vi "Logger.End.vi"(8 "error in":errorcluster, 10 "SeqData":T1={"BeginTS"=timestamp(0 s since 1904-01-01), "EndTS"=timestamp(0 s since 1904-01-01), "State"=enum."Init", "Status.Work"=enum."-", "Status.Process"=enum."-", "Status.Home"=enum."-", "Status.Wabco"=enum."-", "Status.Client"=enum."-", "BreakReason"=enum."OK container", "BreakSource"=enum."-", "DoorLock"=FALSE, "Status.Prod"=[], "UserAction"={"Stop"=FALSE, "Pause"=FALSE, "Next"=FALSE}, "UserData"={"GuiMode"=enum."Process", "Test"={"IgnoreResults"=FALSE, "IgnoreImages"=FALSE, "ServiceMode"=FALSE}, "ContinueOrder"=FALSE}, "Error"={"status"=FALSE, "code"=0, "source"=""}, "Code"={"Ready"=FALSE, "DoubleOrder"=FALSE, "OrderDone"=FALSE, "AllowSingleSlot"=FALSE, "CheckDM"=FALSE, "ThresholdA"=0, "ThresholdB"=0, "Plate"=enum."Wabco", "ImgPath"=path "", "Variant"={"State"=enum."Init", "ImgPath"=path "", "WabcoPlate"="", "WabcoProduct"="", "ClientProduct"="", "ClientPlate"="", "TotalQuantity"=0, "OrderQuantity"=0, "Serial"=0, "Wabco"={"LaserJob"="", "AdditionalTxt"="037", "FactoryCode"="", "RevID"=0, "ForkID"=0, "FailuresLimit"=0, "GlobalCnt"=0, "ScannerProgram"=0, "SerialFormat"=enum."6 dig", "CoordA"={"X"=0.0, "Y"=0.0, "Angle"=0.0}, "CoordB"={"X"=0.0, "Y"=0.0, "Angle"=0.0}, "DMCconfig"=0}, "Client"={"LaserJob"="", "AdditionalTxt"="", "FactoryCode"="037", "RevID"=0, "ForkID"=0, "FailuresLimit"=0, "GlobalCnt"=0, "ScannerProgram"=0, "SerialFormat"=enum."6 dig", "CoordA"={"X"=0.0, "Y"=0.0, "Angle"=0.0}, "CoordB"={"X"=0.0, "Y"=0.0, "Angle"=0.0}, "DMCconfig"=0}}}, "Rotations"=0, "ProdIdx"=0, "ProdDone"=[], "PrintedSerials-Wabco"=[], "PrintedSerials-Client"=[], "Counters-Wabco"={"Expected"=0, "Done"=0, "OK"=0, "NOK"=0, "NOKlimit"=0, "Part"=0, "PartOK"=0}, "Counters-Client"={"Expected"=0, "Done"=0, "OK"=0, "NOK"=0, "NOKlimit"=0, "Part"=0, "PartOK"=0}}, 11 "Refnum in":refnum<k34>) -> (0 "error out":errorcluster, 3 "File path":path)   [LabVIEW 2016]
uses:
  Sequence/Sequence.Data.ctl
  Sequence/Sequence.State.ctl
  Sequence/Sequence.Step.Status.ctl
  Sequence/Sequence.Test.BreakReason.ctl
  Sequence/Sequence.Test.BreakSource.ctl
  Sequence/Sequence.Test.Status.ctl
  Sequence/Sequence.Slot.StatusData.ctl
  Sequence/Sequence.Test.Unload.Status.ctl
  Sequence/Sequence.Prod.StatusData.ctl
  Sequence/Sequence.UserActions.ctl
  Sequence/Sequence.UserData.ctl
  Sequence/Sequence.MainMode.ctl
  Gui/MainGui.TestOptions.ctl
  Sequence/Sequence.Code.Sets.ctl
  Sequence/Sequence.PlateType.ctl
  Logger.Variant.Sets.ctl
  Station/Station.Changeover.State.vi
  Station/Station.Plate.Properties.ctl
  Sequence/Sequence.Code.SerialFormat.ctl
  Drivers/V7310/LowLevel/V7310.Job.Sets.ctl
  Sequence/Sequence.Counters.ctl
  tools/EventLog/EventLog.EventSource.ctl
  tools/Translator/Translator.Message.ctl
  tools/EventLog/EventLog.New(single).vi
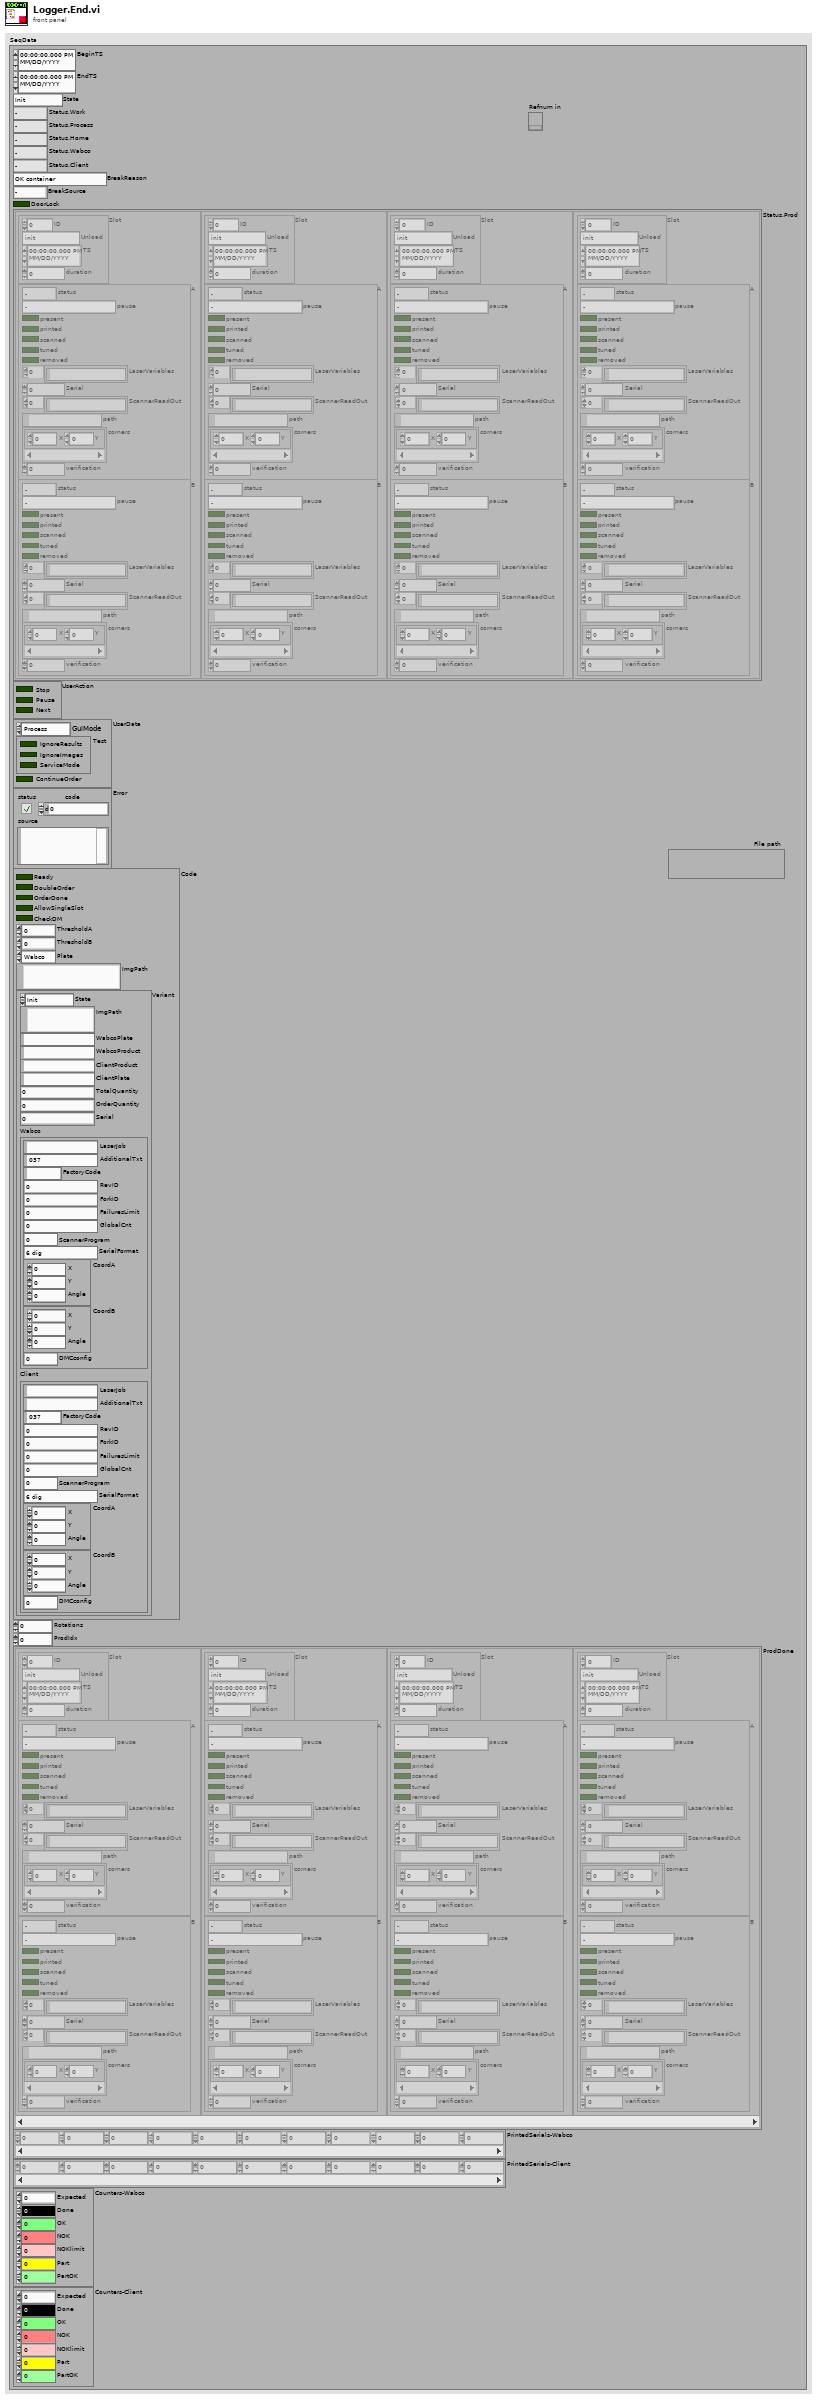
[diagram p1: front panel]
types:
  T1 = typedef "Sequence.Data.ctl" = cluster{"BeginTS":timestamp, "EndTS":timestamp, "State":T2, "Status.Work":T3, "Status.Process":T3, "Status.Home":T3, "Status.Wabco":T3, "Status.Client":T3, "BreakReason":T4, "BreakSource":T5, "DoorLock":bool, "Status.Prod":T6[], "UserAction":T10, "UserData":T11, "Error":errorcluster, "Code":T14, "Rotations":i32, "ProdIdx":i32, "ProdDone":T6[], "PrintedSerials-Wabco":i32[], "PrintedSerials-Client":i32[], "Counters-Wabco":T21, "Counters-Client":T21}
  T2 = typedef "Sequence.State.ctl" = enum16{"Init", "Idle", "Home", "Work", "Run", "Pause"}
  T3 = typedef "Sequence.Step.Status.ctl" = enum16{"-", "Pending", "Running", "Skipped", "Passed", "Failed", "Done", "Error", "Aborted", "Stopped"}
  T4 = typedef "Sequence.Test.BreakReason.ctl" = enum16{"-", "NOK container", "OK container", "Rev empty", "Rev missing", "Rev wrong", "Fork missing", "Fork wrong", "NOK limit", "Unload failure", "Single slot", "Part done", "Err: Prod move work", "Err: Prod move home", "Err: Prod lift work", "Err: Prod lift home", "Err: Prod Arm Work", "Err: Prod Arm NOK", "Err: Prod Arm OK", "Err: Prod NOK suck", "Err: Prod NOK drop", "Err: Prod OK missing", "Err: Prod OK suck", "Err: Prod OK drop"}
  T5 = typedef "Sequence.Test.BreakSource.ctl" = enum16{"-", "A", "B", "A/B"}
  T6 = typedef "Sequence.Test.Status.ctl" = cluster{"Slot":T7, "A":T9, "B":T9}
  T7 = typedef "Sequence.Slot.StatusData.ctl" = cluster{"ID":i32, "Unload":T8, "TS":timestamp, "duration":u32}
  T8 = typedef "Sequence.Test.Unload.Status.ctl" = enum16{"init", "check NOK", "check OK", "wait on NOK", "wait on OK", "wait on Unload", "done"}
  T9 = typedef "Sequence.Prod.StatusData.ctl" = cluster{"status":T3, "pause":T4, "present":bool, "printed":bool, "scanned":bool, "tuned":bool, "removed":bool, "LaserVariables":string[], "Serial":i32, "ScannerReadOut":string[], "path":path, "corners":cluster{"X":i32, "Y":i32}[], "verification":u8}
  T10 = typedef "Sequence.UserActions.ctl" = cluster{"Stop":bool, "Pause":bool, "Next":bool}
  T11 = typedef "Sequence.UserData.ctl" = cluster{"GuiMode":T12, "Test":T13, "ContinueOrder":bool}
  T12 = typedef "Sequence.MainMode.ctl" = enum16{"Process", "Base", "Order", "Manual", "Logs", "Results", "Stats", "DMC Config"}
  T13 = typedef "MainGui.TestOptions.ctl" = cluster{"IgnoreResults":bool, "IgnoreImages":bool, "ServiceMode":bool}
  T14 = typedef "Sequence.Code.Sets.ctl" = cluster{"Ready":bool, "DoubleOrder":bool, "OrderDone":bool, "AllowSingleSlot":bool, "CheckDM":bool, "ThresholdA":u8, "ThresholdB":u8, "Plate":T15, "ImgPath":path, "Variant":T16}
  T15 = typedef "Sequence.PlateType.ctl" = enum16{"Wabco", "Client"}
  T16 = typedef "Logger.Variant.Sets.ctl" = cluster{"State":T17, "ImgPath":path, "WabcoPlate":string, "WabcoProduct":string, "ClientProduct":string, "ClientPlate":string, "TotalQuantity":u16, "OrderQuantity":u16, "Serial":i32, "Wabco":T18, "Client":T18}
  T17 = typedef "Station.Changeover.State.vi" = enum16{"Init", "Scaning", "NOK", "Wait for ack", "Ready"}
  T18 = typedef "Station.Plate.Properties.ctl" = cluster{"LaserJob":string, "AdditionalTxt":string, "FactoryCode":string, "RevID":u8, "ForkID":u8, "FailuresLimit":u16, "GlobalCnt":i32, "ScannerProgram":u8, "SerialFormat":T19, "CoordA":T20, "CoordB":T20, "DMCconfig":i32}
  T19 = typedef "Sequence.Code.SerialFormat.ctl" = enum8{"", "6 dig", "7 dig"}
  T20 = typedef "V7310.Job.Sets.ctl" = cluster{"X":dbl, "Y":dbl, "Angle":dbl}
  T21 = typedef "Sequence.Counters.ctl" = cluster{"Expected":u16, "Done":u16, "OK":u16, "NOK":u16, "NOKlimit":u16, "Part":u16, "PartOK":u16}
  T22 = typedef "Translator.Message.ctl" = enum16{"-", "Event confirmed", "Log out", "Log in", "Shutdown", "Cancel", "Start", "Begin time", "End time", "Duration", "Service Mode", "Ignore Results", "Serial Format", "On", "Off", "OK", "NOK", "NOK %s", "Home", "Work", "Close", "Open", "In progress...", "Missing", "Empty", "Hardware failure", "Initial", "Default", "Total", "Out of range", "Free disk space is below 1GB - contact technician", "Error %d >> %s", "Error %d >> %s >> %s", "Msg %d >> %s", "Laser msg %d %s", "Laser cmd error %s %d", "Laser cmd failed %s", "Laser cmd warning %s", "Laser disconnected", "Laser status %s", "Laser already started", "Laser job unkonwn %s", "Laser job missing %s", "Laser job select failure %s", "Unable to start laser printing (%s)", "Unable to stop laser printing (%s)", "Laser marking aborted", "Laser marking timeout", "Unable to reset Laser Interlock (%s)", "Unable to trigger Laser. Laser not ready (%s)", "Laser job '%s' coordinates not configured", "Starting %s", "Quitting %s", "Configured", "Initializing", "Quitting", "Loading", "Loaded %d results", "Loaded %d events", "Running", "Stopped", "Summary", "Laser", "Do you want to continue?", "Do you want to delete the configuration?", "The configuration is being used by an order. Unable to delete!", "Press confirm button", "Station is not based. Do you want to exit?", "Station requires changeover. Do you want to run the test?", "Test options are not set as default. Do you want to continue?", "Formatting of WabcoNo is disabled. Do you want to continue?", "Product not detected. Do you want to continue?", "Product scan failed. Do you want to continue?", "Calibration", "Log out?", "System", "All", "IDLE", "Translating...%s", "Not found", "Alarm %s", "Run", "Skip", "Abort", "Repeat", "Please wait...", "Database disconnected", "Database disconnected - changeover disabled!", "Login to database successful", "Login to database failed: %d; %s", "Unable to check the product status of reference %d - database disconnected", "Unable to set the product status of reference %d - database disconnected", "Variant file backup %s", "Read variant (%s)", "Result", "Station armed!", "Station requires changeover!", "Select reference number...", "EMERGENCY BUTTON - press Control button", "EMERGENCY DOOR - press Control button", "Resetting Emergency...", "Unable to reset safety circuit - Emergency Button pressed", "Unable to reset safety circuit - Emergency Side Door open", "Station not based", "Station based", "Station not empty", "Station basing...", "No order", "Press Start to begin new order", "Scanning new order", "Order NOK. Correct or scan again", "Order OK. Press Accept", "Order ready", "Revolver incorrect", "Fork incorrect", "Revolver missing", "Revolver empty", "Container missing", "Offline results", "Offline statistics", "Updating statistics %.1f %%", "DMC Configurator", "Door open", "Close the front door", "Press start button", "Done. Open the front door", "Running...", "Running...%.1f %%", "Pause %s", "Pause %s. NOK container missing", "Pause %s. OK container missing", "Pause %s. Revolver empty", "Pause %s. Revolver missing", "Pause %s. Revolver incorrect", "Pause %s. Fork missing", "Pause %s. Fork incorrect", "Pause %s. Too many failures", "Pause %s. Unloading failure", "Pause %s. One slot is not working", "Pause %s. Part order is done. Empty OK container", "Pause %s. Unable to move product to slot", "Pause %s. Unable to move back product pusher", "Pause %s. Unable to lift product", "Pause %s. Unable to move back product lifter", "Pause %s. Unable to move product arm to Work", "Pause %s. Unable to move product arm to NOK", "Pause %s. Unable to move product arm to OK", "Pause %s. Unable to unsuck the NOK product", "Pause %s. Unable to drop the NOK product", "Pause %s. Product OK missing", "Pause %s. Unable to unsuck the OK product", "Pause %s. Unable to drop the OK product", "Stopping...", "File '%s' is missing", "File '%s' is broken", "File '%s' is running", "Log file started (%s)", "Log file ended (%s)", "Log file stopped (%s)", "Log file ignored (%s)", "Log file exported (%s)", "Log file export failed (%s)", "Wrong serial number in log file", "Wrong reference number in log file", "Test steps are missing", "%s = %.3f", "Process param '%s' not found in DB", "Process param '%s' wrong order", "Process param '%s' value %.3f out of limits (%.3f; %.3f)", "Step%d param '%s' not found in DB", "Step%d param '%s' wrong order", "Step%d param '%s' value %.3f out of limits (%.3f; %.3f)", "Step%d EV '%s' not found in DB", "Step%d EV '%s' wrong order", "\"%s\" not found in DB", "\"%s\" wrong order", "\"%s\" value %.3f out of limits (%.3f; %.3f)", "\"%s\" not found in software", "Process init (%s)", "Process started", "Process restarted", "Process run", "Process done", "Process done - remove OK container", "Process aborted", "Process aborted at work", "Process aborted at home", "Process error", "Process error at home", "Process error at work", "Process close", "Process pause", "Process continue", "Process door open", "Process door close", "Process pause at slot %s due to %s", "Select plate from the order to process", "Do you want to start the process?", "Do you want to continue the process?", "There is unfinished order. Do you want to put the new order?", "Product %s %d OK", "Product %s %d NOK", "Unable to unload the slot %s. Product missing in the slot", "Unable to unload the slot %s. Product already in the arm", "Unable to accept the product as OK. Product missing in slot %s", "Unable to accept the product as OK. Product could not drop into the container at slot %s", "Unable to accept the product as NOK. Product could not drop into the container at slot %s", "Scan failed. Error %s", "Scan failed. Scanner disconnected", "Scan failed. Wrong Wabco number %d, limit (%d,%d)", "Scan failed. Wrong serial number %d, limit (%d,%d)", "Scan failed. Wrong date %d, limit (%d,%d)", "Scan failed. Wrong product wabco number %d (expected %d)", "Scan failed. Wrong product serial number %d (expected > 0)", "Scan OK %s", "Scan failed. Unable to determine table position (%s)", "Scan failed. Timeout", "Tune failed. Scanner disconnected", "Tune failed. Timeout", "%s = %d", "%s = %d->%d", "Unable to set %s = %.2f - Air Pressure Inside off", "Unable to set digital output '%s' = %d", "Unable to activate air pressure inside - timeout", "Unable to activate air pressure inside - aborted", "Unable to switch on Air Main Valve - Air Pressure Inlet off", "Unable to switch on Air Main Valve - Door open", "Unable to switch off Air Main Valve - timeout", "Unable to switch off Air Main Valve - aborted", "Unable to rotate Table - timeout", "Unable to rotate Table - aborted", "Unable to rotate Table - Product Move not in Home position", "Unable to rotate Table - Air Pressure Inside off", "Unable to rotate Table - Product Lift A not in Home position", "Unable to rotate Table - Product Lift B not in Home position", "Unable to rotate Table - unlock before movement timeout", "Unable to rotate Table - lock after movement timeout", "Unable to move Table Lock to %s position - timeout", "Unable to move Table Lock to %s position - aborted", "Unable to move Table Lock to %s position - Air Pressure Inside off", "Unable to move Table Lock to %s position - Table not in position", "Unable to move Product Lift A to %s position - timeout", "Unable to move Product Lift B to %s position - timeout", "Unable to move Product Lift A to %s position - aborted", "Unable to move Product Lift B to %s position - aborted", "Unable to move Product Lift A to %s position - Air Pressure Inside off", "Unable to move Product Lift B to %s position - Air Pressure Inside off", "Unable to move Product Lift A to %s position - Table not locked", "Unable to move Product Lift B to %s position - Table not locked", "Unable to move Product Lift A to %s position - Product Arm not in Work position", "Unable to move Product Lift B to %s position - Product Arm not in Work position", "Unable to set Product Suction Gripper %s to %s - timeout", "Unable to set Product Suction Gripper %s to %s - aborted", "Unable to set Product Suction Gripper %s to %s - Air Pressure Inside off", "Unable to set Product Suction Gripper %s to %s - Table slot unkown", "Unable to move Product Arm to %s position - timeout", "Unable to move Product Arm to %s position - aborted", "Unable to move Product Arm to %s position - Air Pressure Inside off", "Unable to move Product Arm to %s position - Product Lift A not in Home position", "Unable to move Product Arm to %s position - Product Lift B not in Home position", "Unable to move Product to %s position - timeout", "Unable to move Product to %s position - aborted", "Unable to move Product to %s position - Air Pressure Inside off", "Unable to move Product to %s position - Table not in position"}
  T23 = typedef "EventLog.EventSource.ctl" = enum16{"All", "Gui", "Ref", "File", "Arch", "Seq", "CPX", "DB", "Laser", "Scan.P", "Scan.O"}
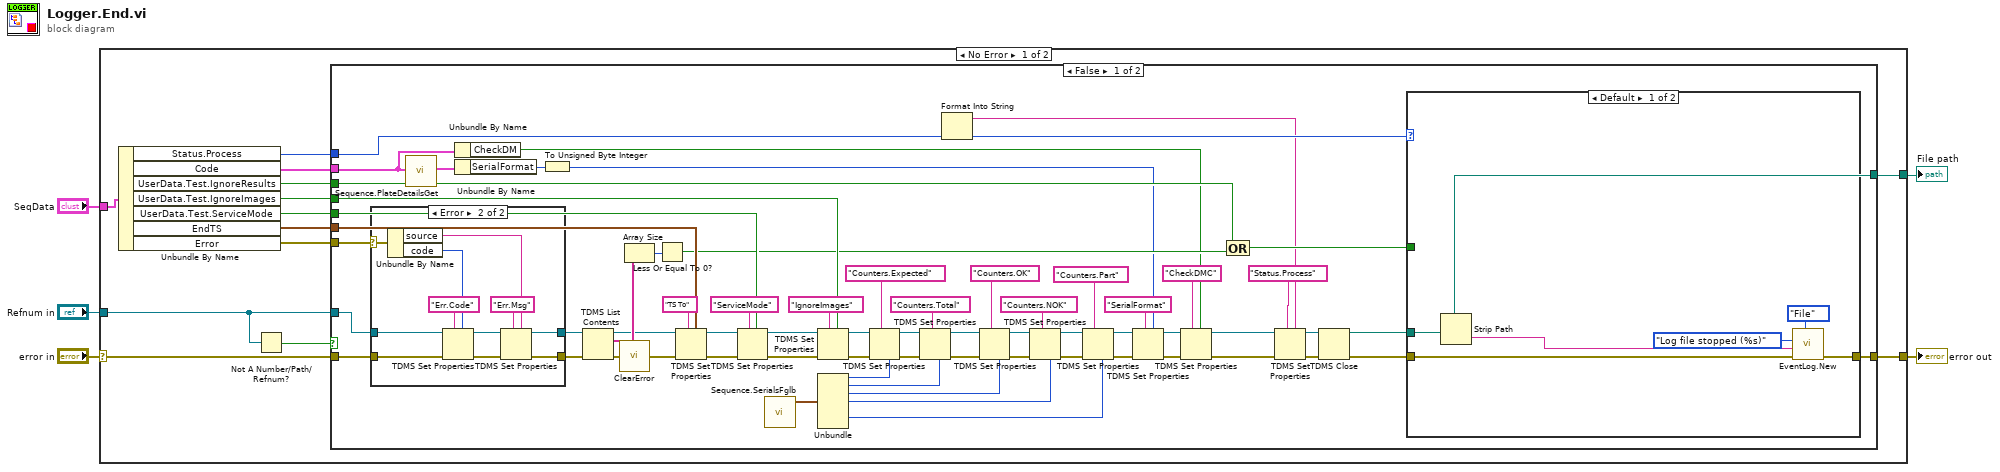
[diagram p0: block diagram]
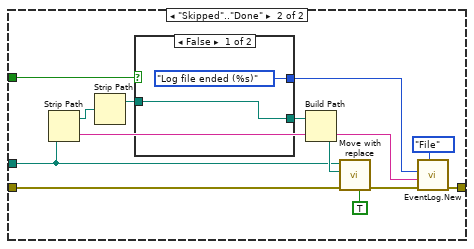
[diagram p3: hidden frame]
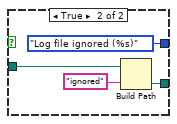
[diagram p4: hidden frame]
diagram:
  n1 = case shown="No Error" "error in" {
    selector: "error in" -> [w18 w123]
    tunnel: [w17 w123] -> w5
    tunnel: "Refnum in" -> [w14 _]
    tunnel: "SeqData" -> [w13 _]
    tunnel: [w7 _] -> w1
    frame No Error {
      n2 = Unbundle By Name(w13) -> ("Status.Process"=w6:T3, "Code"=w8:T14, "UserData.Test.IgnoreResults"=w9:bool, "UserData.Test.IgnoreImages"=w10:bool, "UserData.Test.ServiceMode"=w11:bool, "EndTS"=w12:timestamp, "Error"=w15:errorcluster)
      n3 = Not A Number/Path/Refnum?(number/path/refnum=w14) -> (NaN/Path/Refnum?=w16:bool)
      n4 = case shown="False" w16 {
        tunnel: w18 -> [w80 w122]
        tunnel: w14 -> [w78 _]
        tunnel: w12 -> [w73 _]
        tunnel: [w76 w122] -> w17
        tunnel: w15 -> [w81 _]
        tunnel: w11 -> [w71 _]
        tunnel: w10 -> [w70 _]
        tunnel: w9 -> [w67 _]
        tunnel: w8 -> [w20 _]
        tunnel: [w28 _] -> w7
        tunnel: w6 -> [w24 _]
        frame False {
          n5 = case shown="Error" w81 {
            selector: w81 -> [_ w93]
            tunnel: w80 -> [w85 w95]
            tunnel: [w85 w89] -> w79
            tunnel: w78 -> [w84 w94]
            tunnel: [w84 w88] -> w77
            frame No Error {
            }
            frame Error {
              n6 = Unbundle By Name(w93) -> ("source"=w86:string, "code"=w92:i32)
              n7 = TDMS Set Properties(5:w92, 7:"Err.Code", 8:w95, 11:w94) -> (0:w90:errorcluster, 3:w87:refnum<k34>)  [unwired: 2 in, 2 out]
              n8 = TDMS Set Properties(5:w86, 7:"Err.Msg", 8:w90, 11:w87) -> (0:w89:errorcluster, 3:w88:refnum<k34>)  [unwired: 2 in, 2 out]
            }
          }
          n9 = call "Sequence.PlateDetailsGet.vi"("Code in"=w20) -> ("PlateDetails"=w37:T18)  [unwired: 9 in, 1 out]
          n10 = Unbundle By Name(w20) -> ("CheckDM"=w19:bool)
          n11 = Unbundle By Name(w37) -> ("SerialFormat"=w35:T19)
          n12 = To Unsigned Byte Integer(number=w35) -> (unsigned 8bit integer=w34:u8)
          n13 = TDMS List Contents(4:w79, 7:w77) -> (0:w72:errorcluster, 2:w83:string[], 3:w75:refnum<k34>)  [unwired: 1 in, 1 out]
          n14 = call <vilib>:"ClearError.vi"("error in (no error)"=w72) -> ("error out"=w74:errorcluster)
          n15 = Array Size(array=w83) -> (size(s)=w82:i32)
          n16 = Less Or Equal To 0?(x=w82) -> (x <= 0?=w69:bool)
          n17 = TDMS Set Properties(5:w73, 7:"TS To" ("format string"), 8:w74, 11:w75) -> (0:w60:errorcluster, 3:w61:refnum<k34>)  [unwired: 2 in, 2 out]
          n18 = TDMS Set Properties(5:w71, 7:"ServiceMode", 8:w60, 11:w61) -> (0:w59:errorcluster, 3:w62:refnum<k34>)  [unwired: 2 in, 2 out]
          n19 = call "Sequence.SerialsFglb.vi"() -> ("Counters out"=w39:T21)  [unwired: 7 in, 4 out]
          n20 = TDMS Set Properties(5:w70, 7:"IgnoreImages", 8:w59, 11:w62) -> (0:w54:errorcluster, 3:w53:refnum<k34>)  [unwired: 2 in, 2 out]
          n21 = Unbundle(w39) -> ("Expected"=w52:u16, "Done"=w51:u16, "OK"=w44:u16, "NOK"=w43:u16, "Part"=w38:u16)  [unwired: 2 out]
          n22 = TDMS Set Properties(5:w52, 7:"Counters.Expected", 8:w54, 11:w53) -> (0:w58:errorcluster, 3:w57:refnum<k34>)  [unwired: 2 in, 2 out]
          n23 = TDMS Set Properties(5:w51, 7:"Counters.Total", 8:w58, 11:w57) -> (0:w46:errorcluster, 3:w45:refnum<k34>)  [unwired: 2 in, 2 out]
          n24 = Format Into String(w24) -> (resulting string=w23:string)  [unwired: 3 in, 1 out]
          n25 = TDMS Set Properties(5:w44, 7:"Counters.OK", 8:w46, 11:w45) -> (0:w47:errorcluster, 3:w48:refnum<k34>)  [unwired: 2 in, 2 out]
          n26 = TDMS Set Properties(5:w43, 7:"Counters.NOK", 8:w47, 11:w48) -> (0:w40:errorcluster, 3:w41:refnum<k34>)  [unwired: 2 in, 2 out]
          n27 = TDMS Set Properties(5:w38, 7:"Counters.Part", 8:w40, 11:w41) -> (0:w33:errorcluster, 3:w32:refnum<k34>)  [unwired: 2 in, 2 out]
          n28 = TDMS Set Properties(5:w34, 7:"SerialFormat", 8:w33, 11:w32) -> (0:w30:errorcluster, 3:w29:refnum<k34>)  [unwired: 2 in, 2 out]
          n29 = TDMS Set Properties(5:w19, 7:"CheckDMC", 8:w30, 11:w29) -> (0:w26:errorcluster, 3:w25:refnum<k34>)  [unwired: 2 in, 2 out]
          n30 = Compound Arithmetic op=OR(w67, w69) -> (w66:bool)
          n31 = TDMS Set Properties(5:w23, 7:"Status.Process", 8:w26, 11:w25) -> (0:w21:errorcluster, 3:w22:refnum<k34>)  [unwired: 2 in, 2 out]
          n32 = TDMS Close(8:w21, 11:w22) -> (0:w68:errorcluster, 3:w28:path)
          n33 = case shown="Default" w24 {
            tunnel: [w100 w115] -> w76
            tunnel: w68 -> [w101 w108]
            tunnel: w66 -> [_ w104]
            tunnel: w28 -> [w98 w103]
            frame Default {
              n34 = Strip Path(path=w98) -> (name=w97:string)  [unwired: 1 out]
              n35 = call-poly "EventLog.New.vi"("Source (All)"=EventLog.EventSource."File" ("Source (App)"), "error in (no error)"=w101, "Arg"=w97, "Message (-)"=Translator.Message."Log file stopped (%s)") -> ("error out"=w100:errorcluster)  [unwired: 6 in, 1 out]
            }
            frame "Skipped".."Done" {
              n36 = Strip Path(path=w103) -> (stripped path=w105:path, name=w109:string)
              n37 = Strip Path(path=w105) -> (stripped path=w111:path)  [unwired: 1 out]
              n38 = case shown="False" w104 {
                tunnel: w111 -> [w116 w121]
                tunnel: [w116 w120] -> w107
                tunnel: [Translator.Message."Log file ended (%s)" ("Message (-)") Translator.Message."Log file ignored (%s)" ("Message (-)")] -> w106
                frame False {
                }
                frame True {
                  n39 = Build Path(base path=w121, name or relative path="ignored") -> (appended path=w120:path)
                }
              }
              n40 = Build Path(base path=w107, name or relative path=w109) -> (appended path=w114:path)
              n41 = call "Move with replace.vi"("create parent dirs (F)"=TRUE, "error in (no error)"=w108, "destination path"=w114, "source path"=w103) -> ("error"=w112:errorcluster)  [unwired: 7 in]
              n42 = call-poly "EventLog.New.vi"("Source (All)"=EventLog.EventSource."File" ("Source (App)"), "error in (no error)"=w112, "Arg"=w109, "Message (-)"=w106) -> ("error out"=w115:errorcluster)  [unwired: 6 in, 1 out]
            }
          }
        }
        frame True {
        }
      }
    }
    frame Error {
    }
  }
  "error out" <- w5
  "File path" <- w1
